vi "HW_Acquisition_Stop.vi"(2 "Error In":errorcluster, 3 "VISA resource name in":refnum<visa-resource-name>) -> (0 "Error Out":errorcluster, 1 "VISA resource name out":refnum<visa-resource-name>)   [LabVIEW 2018, in "Tracker.lvlib"]
uses:
  <vilib>/Instr/_visa.llb/VISA Flush IO Buffer Mask.ctl
  Tracker.lvlib
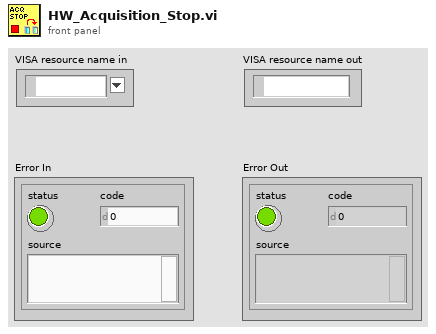
[diagram p1: front panel]
types:
  T1 = typedef "VISA Flush IO Buffer Mask.ctl" = u16
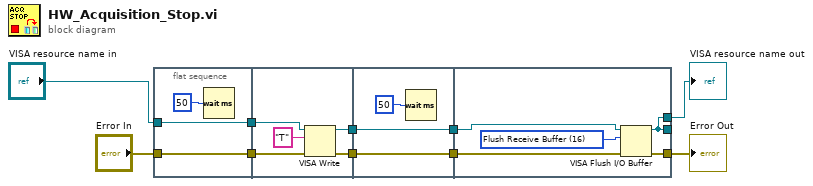
[diagram p0: block diagram]
diagram:
  n1 = flat-sequence {
    tunnel: "VISA resource name in" -> [w12]
    tunnel: "Error In" -> [w13]
    tunnel: [w13] -> w2
    tunnel: [w12] -> w1
    tunnel: [w18] -> w10
    tunnel: [w17] -> w9
    tunnel: w2 -> [w15]
    tunnel: w1 -> [w14]
    tunnel: w10 -> [w20]
    tunnel: w9 -> [w19]
    tunnel: [w20] -> w8
    tunnel: [w19] -> w5
    tunnel: [w22] -> _
    tunnel: w8 -> [w26]
    tunnel: [w24] -> w4
    tunnel: w5 -> [w23]
    tunnel: [w22] -> w3
    frame #0 {
      n2 = Wait (ms)(milliseconds to wait=u32 50) -> ()  [unwired: 1 out]
    }
    frame #1 {
      n3 = VISA Write(VISA resource name=w14, write buffer="T", error in (no error)=w15) -> (VISA resource name out=w18:refnum<visa-resource-name>, error out=w17:errorcluster)  [unwired: 1 out]
    }
    frame #2 {
      n4 = Wait (ms)(milliseconds to wait=u32 50) -> ()  [unwired: 1 out]
    }
    frame #3 {
      w25 = T1 16 items=["Flush Receive Buffer"=16, "Write Transmit Buffer to Device"=32, "Flush Receive Buffer (No I/O)"=64, "Flush Transmit Buffer"=128] ("Mask")
      n5 = VISA Flush I/O Buffer(VISA resource name=w26, mask (16)=w25, error in (no error)=w23) -> (VISA resource name out=w22:refnum<visa-resource-name>, error out=w24:errorcluster)
    }
  }
  "VISA resource name out" <- w3
  "Error Out" <- w4
